vi "Control SCR-1.vi"() -> ()   [LabVIEW 2019]
uses:
  PortConfig.ctl
  <vilib>/Platform/TimedLoop/XDataNode/timing_clust.ctl
  <vilib>/Platform/TimedLoop/XDataNode/nitl_modes.ctl
  <vilib>/Platform/TimedLoop/XDataNode/wakeup.ctl
  <vilib>/Instr/_visa.llb/VISA Configure Serial Port (Instr).vi
  <vilib>/express/express shared/transition.llb/Dynamic To Waveform Array.vi
  <vilib>/express/express signal manip/GetorSetDDTAttributes/Set DDT Attributes/SetT0.vi
  <vilib>/express/express shared/transition.llb/Waveform Array To Dynamic.vi
  <vilib>/express/express signal manip/GetorSetDDTAttributes/Set DDT Attributes/Set DDT Properties.xnode
  <vilib>/platform/TimedLoop/XDataNode/XDataNode.xnode
  <vilib>/Platform/TimedLoop/XDataNode/XDNodeRunTimeDep.lvlib
panel:
  in  "CODIGO DIWO":dbl
  out "Total":dbl format="%#_6f"
  out "Total":dbl(slide) scale=0.0..1500.0
  out "Bobina 4":dbl format="%_3g"
  out "Bobina 0":dbl format="%_3g"
  out "Bobina 8":dbl format="%_3g"
  out "Boolean0":bool
  out "Boolean4":bool
  out "Boolean8":bool
  out "ExeState":string
  out "Next":dbl
  out "ULTIMA":dbl
  in  "Tension en Banco":dbl
  in  "Temperatura en Resistencia":dbl
  out "Temperatura en Bobinas":dbl
  out "E. ECRH":bool
  out "E. Campo":bool
  in  "Stop Button":bool
  out "SECUENCIA FINALIZADA":bool
  out "SECUENCIA INICIADA":bool
  out "Bool0":bool
  out "Bool1":bool
  out "Bool2":bool
  out "Bool3":bool
  out "DESACTIVAR Gas":bool
  out "DESCATIVAR ECRH":bool=TRUE
  out "DESACTIVAR Campo":bool=TRUE
  out "ACTIVAR Diagnosticos":bool=TRUE
  out "ACTIVAR ECRH":bool=TRUE
  out "ACTIVAR Campo":bool=TRUE
  out "Presion":dbl
  out "IG Filament Status":string
  out "Presion Normal":bool
  in  "TD [ms]":dbl
  out "Sistema de Inyeccion de Gas":bool
  out "Diagnosticos":bool
  out "Sistema de ECRH":bool
  out "Sistema de Vacío":bool
  out "Sistema de Potencia":bool
  out "Potencia ECRH":dbl
  out "DESCARGA":bool
  out "SP Fuera de Rango":bool
  out "TC Fuera de Rango":bool
  in  "TC [ms]":dbl
  out "TE1+ TE1 Fuera de Rango":bool
  out "Flujo Aisladores":bool
  in  "Set de Potencia":dbl format="%#_3f"
  out "Fuera de Rango":bool
  out "Rango Normal":bool
  out "P. SET":dbl(knob) scale=0.0..2000.0
  in  "OFF-ON":bool
  out "Boolean":bool
  in  "Secuencia de Descarga":bool
  in  "SP [SCCM]":dbl
  in  "TE1 [ms]":dbl
  in  "TE2 [ms]":dbl
  out "Cuenta C":i32
  out "Iteration Duration A":i64
  out "Iteration Duration B":i64
  out "Iteration Duration C":i64
  out "Iteration Duration D":i64
  out "ACTIVAR Gas":bool
  out "SP1":dbl format="%#_6f"
  out "MFC":dbl format="%#_6f"
  out "Flujo":dbl(knob) scale=0.0..20.0
  out "IG":dbl format="%#_6e"
  out "CG2":dbl format="%#_6e"
  out "CG1":dbl format="%#_6e"
  out "P. Forward":dbl(slide) scale=0.0..1500.0
  out "Forward":dbl format="%#_6f"
  out "P. Reflected":dbl(slide) scale=0.0..1500.0
  out "Reflected":dbl format="%#_6f"
  out "Corriente":dbl(knob) scale=0.0..1000.0
  out "Corriente":dbl format="%#_6f"
  in  "MFC":refnum<visa-resource-name>="COM11"
  in  "IonGauge":refnum<visa-resource-name>="COM12"
  in  "Nombre de Archivo":string="SCR-1_TEST.txt"
  in  "Error In":errorcluster
  out "Cuenta B":i32
  out "Cuenta A":i32
  out "Cuenta D":i32
  out "SECUENCIA":bool caption="Boolean"
  out "INYECCION DE GAS":bool caption="Boolean"
  out "DATOS":bool caption="Boolean"
  out "SEGURIDAD":bool caption="Boolean"
  in  "TG 2":i64=5
  in  "TG 1":i64=5
  # "INDICADORES"
  # "CONFIGURACION"
  # "PARAMETROS DE EXPERIMENTO"
  # "CALENTAMIENTO ECRH"
  # "INYECCION DE GAS"
  # "CAMPO MAGNETICO"
  # "MAGNETRON 2kW"
  # "DISPARO DE DIAGNOSTICOS"
  # "GENERACION DE VACIO"
  # "PARAMETROS INICIALES"
  # "Configuracion"
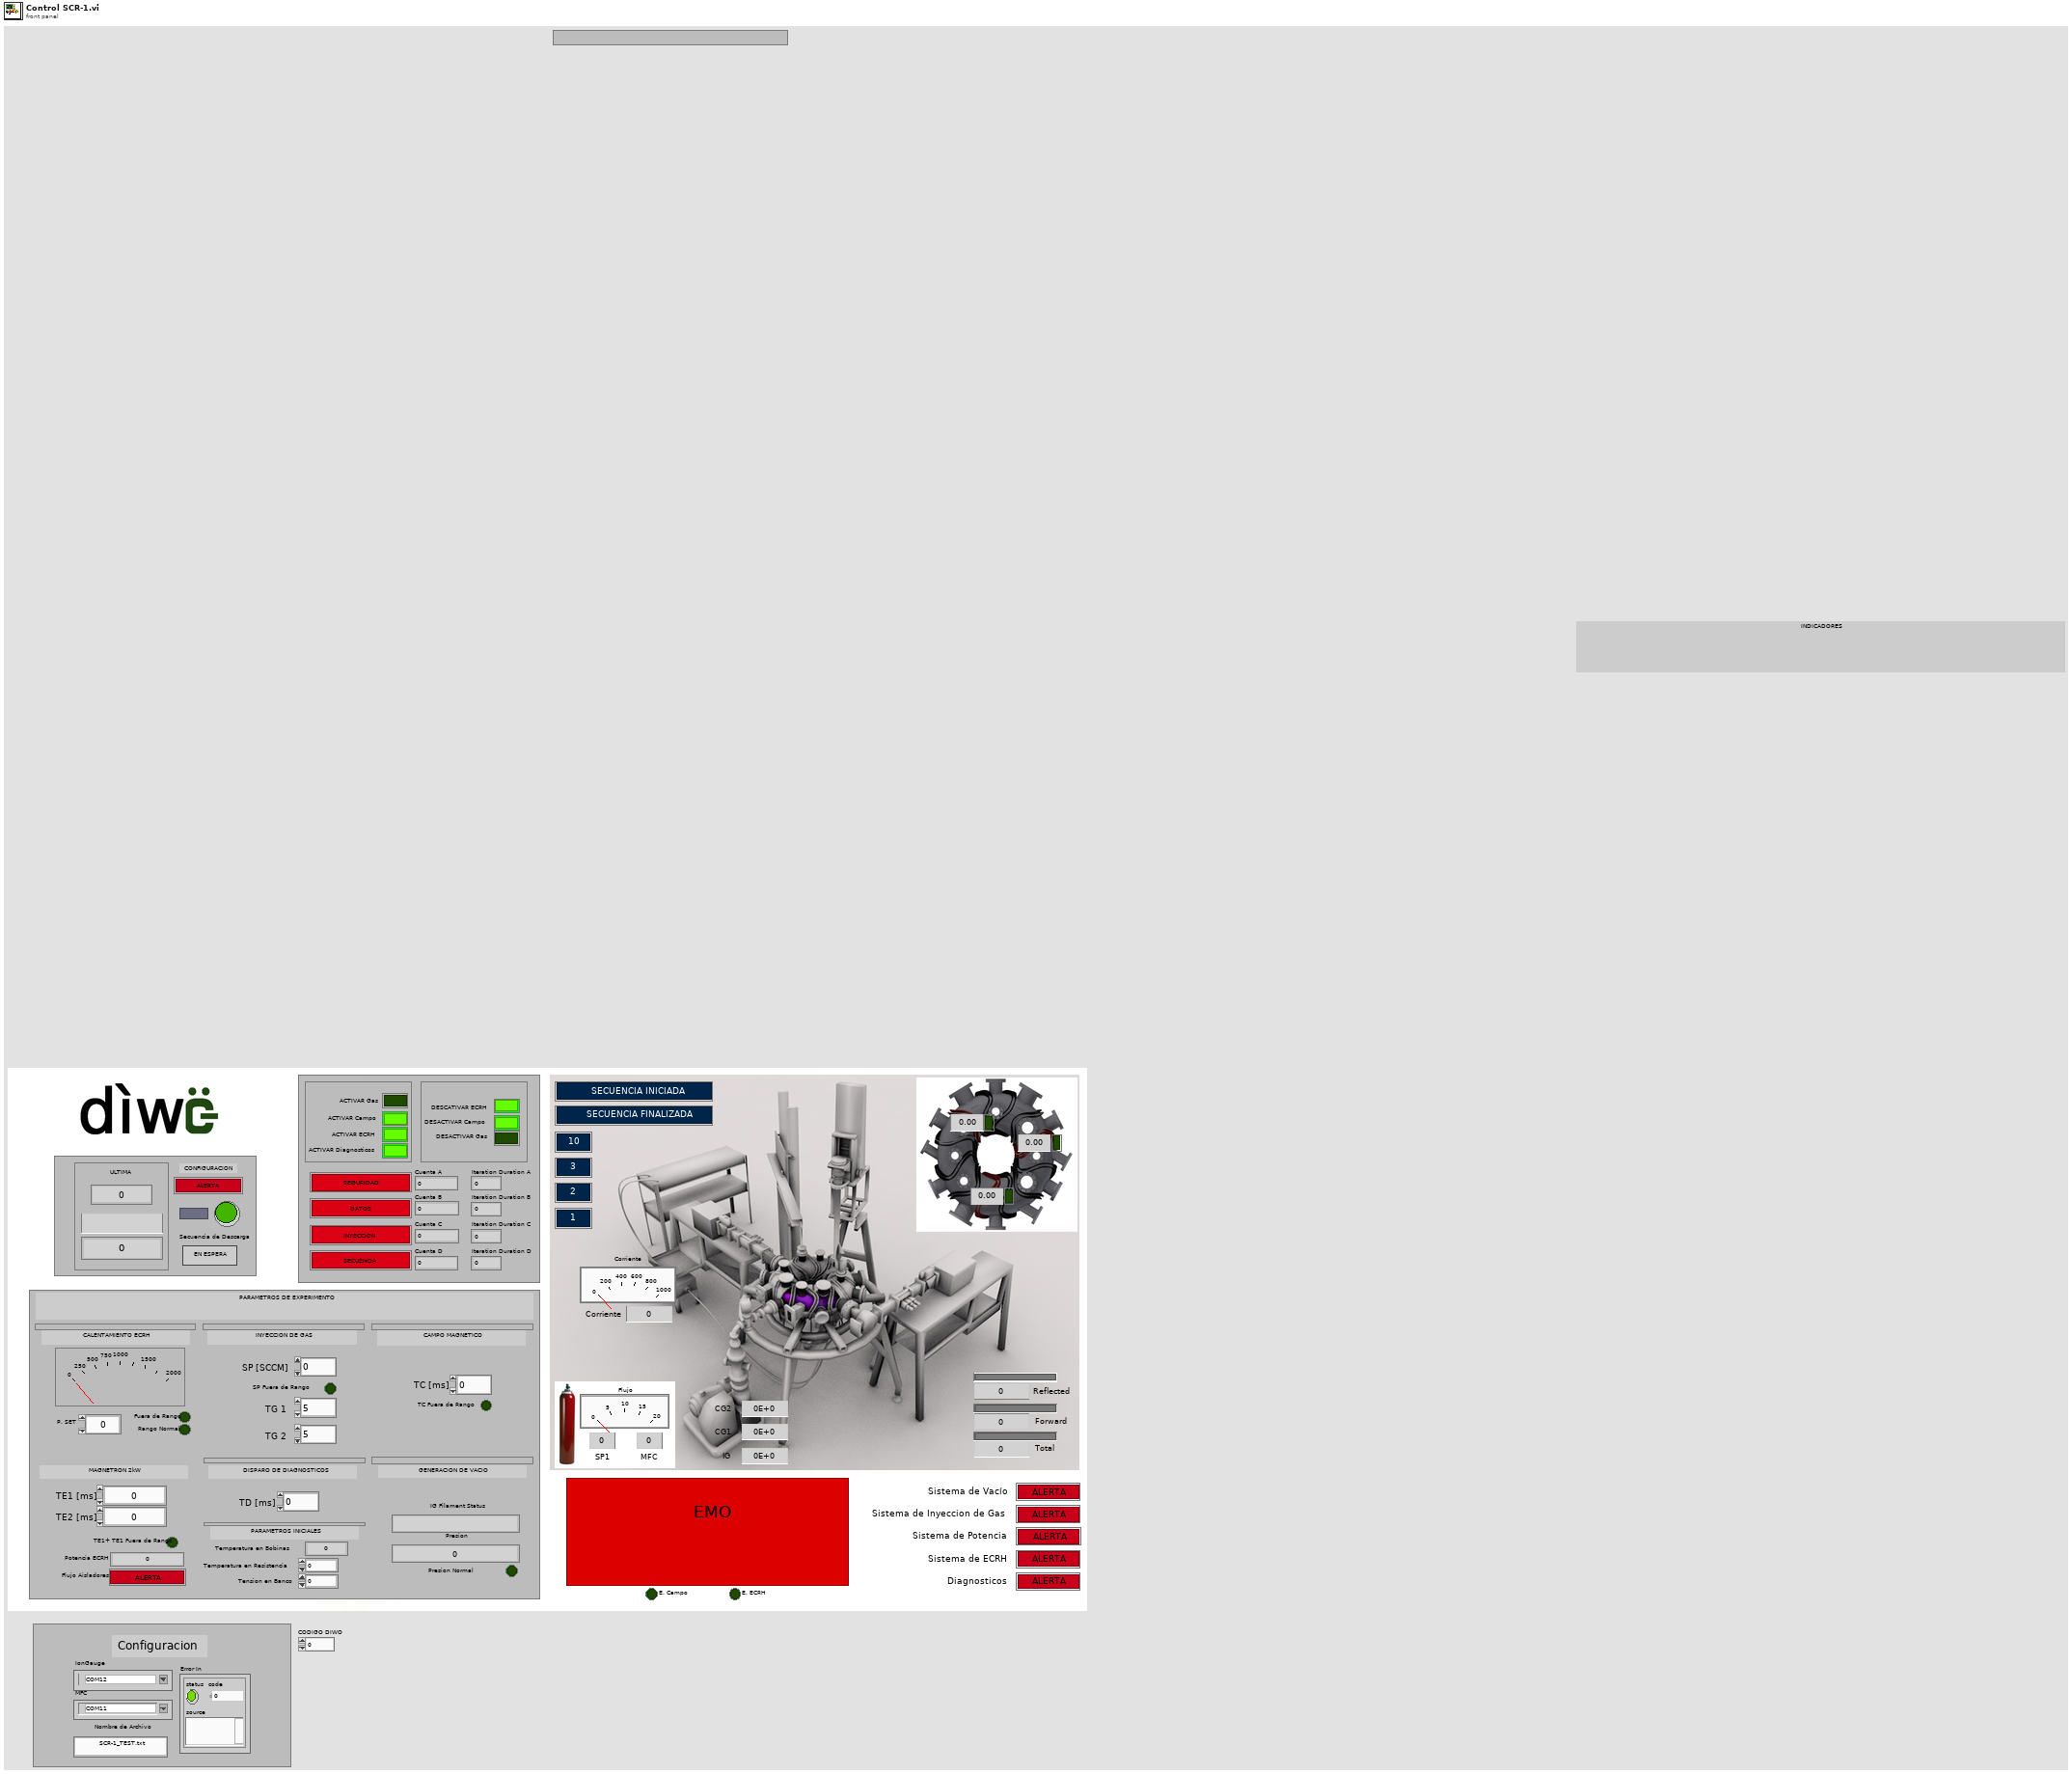
[diagram p1: front panel]
types:
  T1 = typedef "PortConfig.ctl" = cluster{"baud rate":u32, "data bits":u16, "parity":enum16{"None", "Odd", "Even", "Mark", "Space"}, "stop bits":u16}
  T2 = cluster{"VISA resource name out":refnum<visa-resource-name>, "error out":errorcluster, "VISA resource name out":refnum<visa-resource-name>, "error out":errorcluster}
  T3 = cluster{"TD [ms]":dbl, "Set de Potencia":dbl, "TE2 [ms]":dbl, "TE1 [ms]":dbl, "TC [ms]":dbl, "SP [SCCM] ":dbl}
  T4 = typedef "XDNodeRunTimeDep.lvlib/timing_clust.ctl" = cluster{"Expected End [f-1]":u64, "Actual End [f-1]":u64, "Finished Late? [f-1]":bool, "Expected End [i-1]":u64, "Actual End [i-1]":u64, "Finished Late? [i-1]":bool, "Expected Start [i]":u64, "Actual Start [i]":u64, "Expected Start [f]":u64, "Actual Start [f]":u64, "Source Name":string, "Structure Name":string, "Period":i64, "Deadline":i64, "Offset":i64, "Start":i64, "Priority":i32, "Timeout":i32, "Mode":T5, "Wakeup Reason":T6, "Error":errorcluster, "Source Type":string, "Secondary Source Type":string, "Global End Time":u64, "Global Start Time":u64, "Frame Duration":u64, "Iteration Duration":u64, "Assigned CPU":i32, "I/O Scan Engine Mode":u32}
  T5 = typedef "XDNodeRunTimeDep.lvlib/nitl_modes.ctl" = enum32{"No Change", "Process missed periods, maintain original phase", "Discard missed periods, maintain original phase", "Process missed periods, ignore original phase", "Discard missed periods, ignore original phase"}
  T6 = typedef "XDNodeRunTimeDep.lvlib/wakeup.ctl" = enum32{"Normal", "Aborted", "Asynchronous wakeup", "Timing source error", "Timed loop error", "Timeout"}
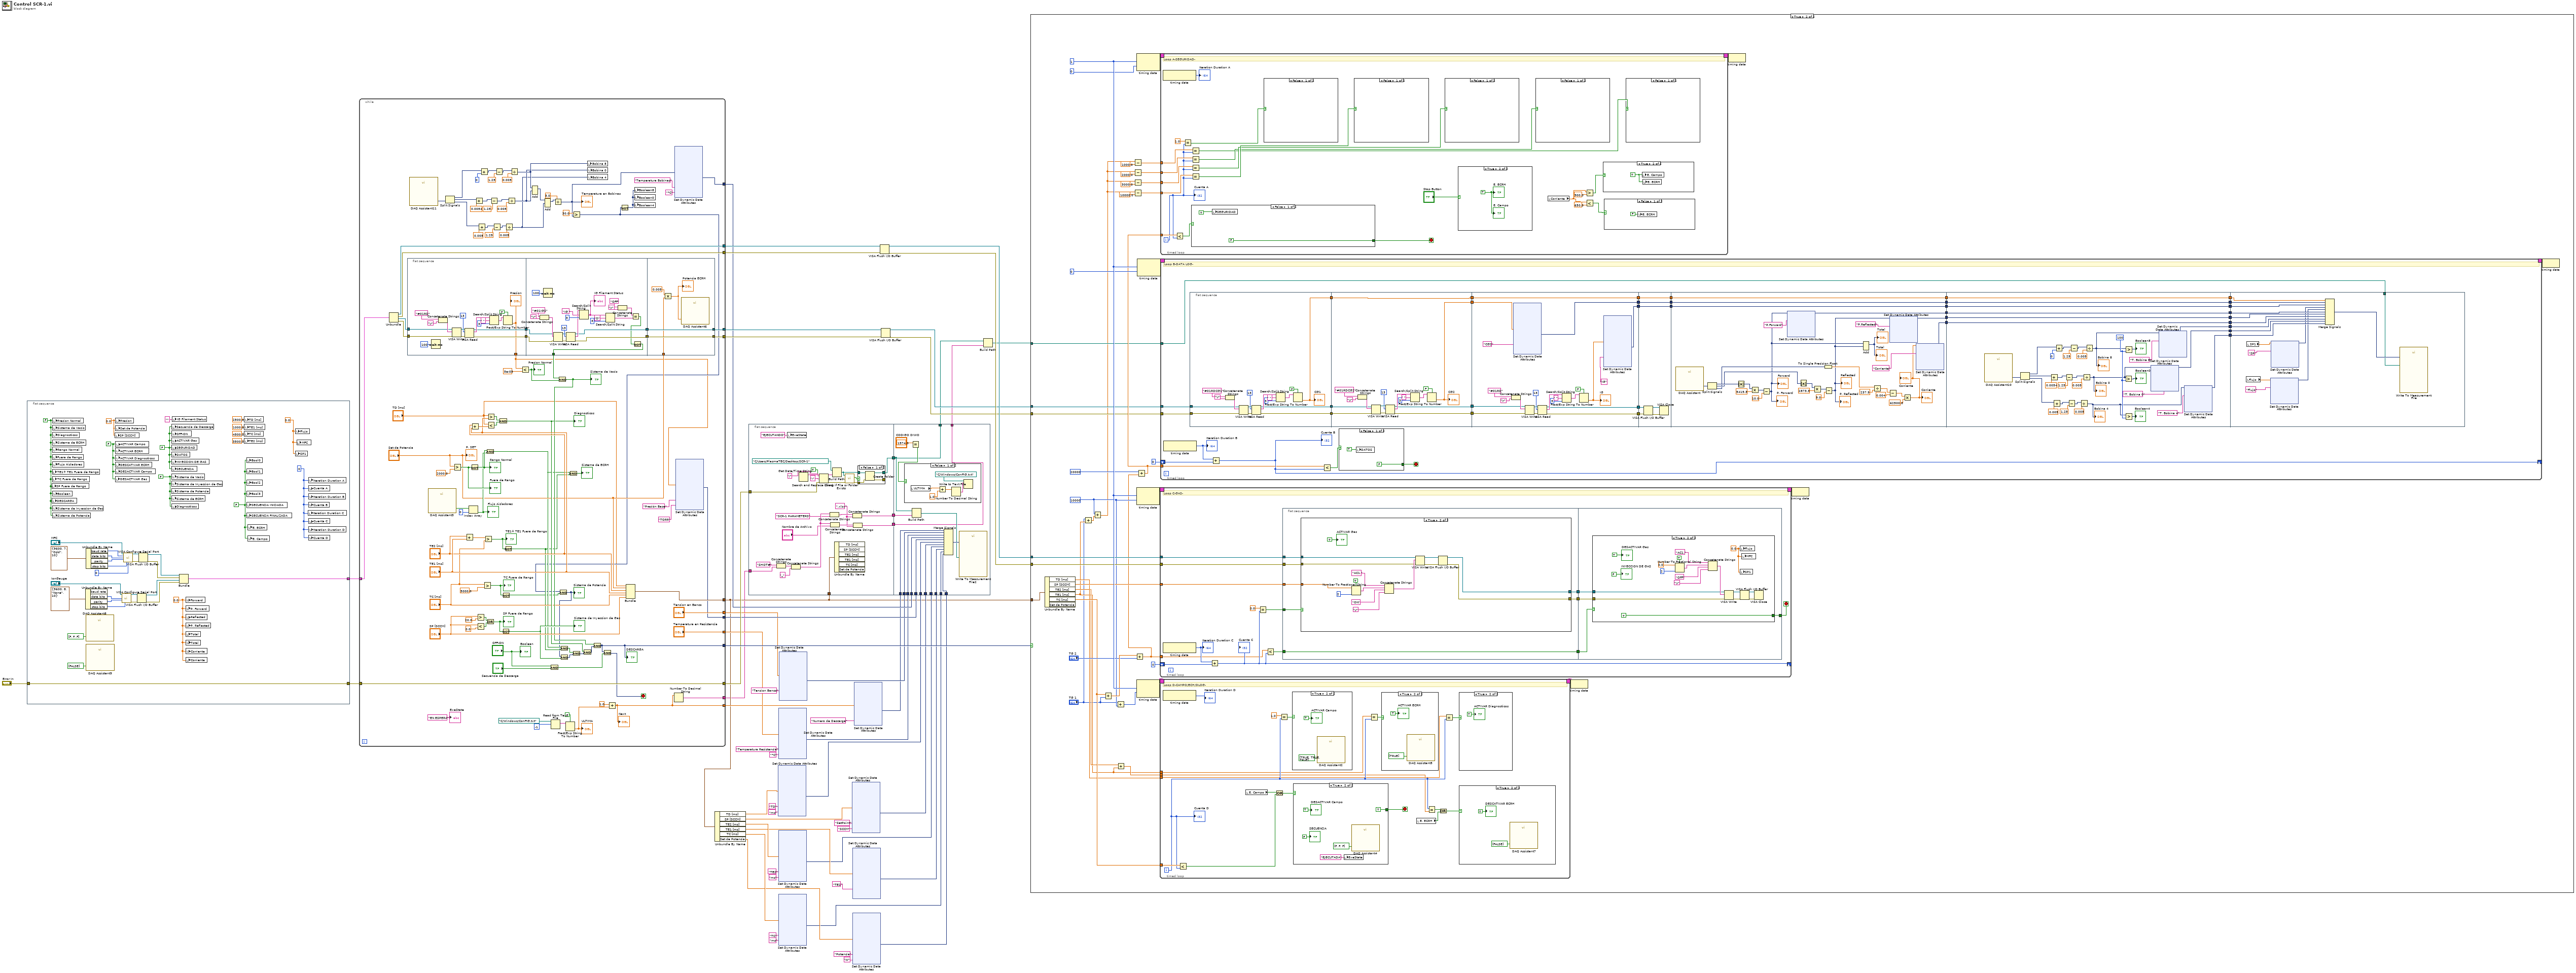
[diagram p0: block diagram]
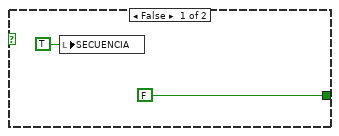
[diagram p9: hidden frame]
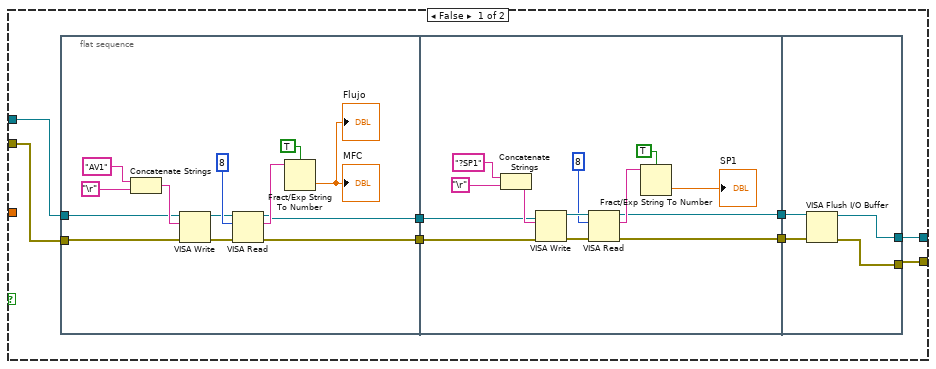
[diagram p10: hidden frame]
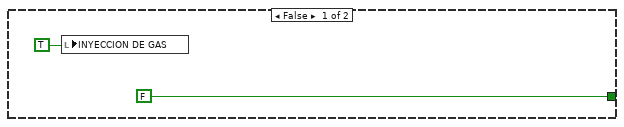
[diagram p11: hidden frame]
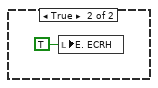
[diagram p12: hidden frame]
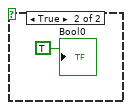
[diagram p15: hidden frame]
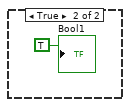
[diagram p16: hidden frame]
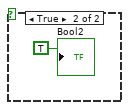
[diagram p17: hidden frame]
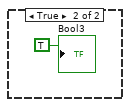
[diagram p18: hidden frame]
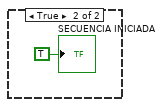
[diagram p19: hidden frame]
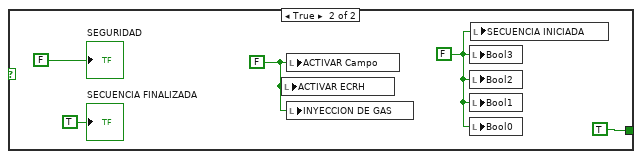
[diagram p20: hidden frame]
diagram:
  n1 = flat-sequence {
    tunnel: [w94] -> w52
    tunnel: "Error In" -> [w94]
    tunnel: [w80] -> w48
    frame #0 {
      w57 = 0.0 ("Forward")
      w62 = 0.0 ("SetPoint")
      w58 = i64 0 ("Iteration Duration C")
      w61 = FALSE ("SECUENCIA INICIADA")
      w63 = FALSE ("CAMPO ON")
      w69 = 0.0 ("Presion")
      w78 = FALSE ("Presion Normal")
      w93 = FALSE ("Sistema de Vacío")
      w64 = FALSE ("SEGURIDAD")
      n2 = local write "SP Fuera de Rango"(w78) -> ()
      n3 = local write "DESCARGA"(w78) -> ()
      n4 = local write "TE1+ TE1 Fuera de Rango"(w78) -> ()
      n5 = local write "TC Fuera de Rango"(w78) -> ()
      n6 = local write "Presion Normal"(w78) -> ()
      n7 = local write "Sistema de Vacío"(w78) -> ()
      n8 = local write "Diagnosticos"(w78) -> ()
      n9 = local write "Sistema de ECRH"(w78) -> ()
      n10 = local write "Rango Normal"(w78) -> ()
      n11 = local write "Fuera de Rango"(w78) -> ()
      n12 = local write "Flujo Aisladores"(w78) -> ()
      n13 = local write "Boolean"(w78) -> ()
      n14 = local write "Sistema de Inyeccion de Gas"(w78) -> ()
      n15 = local write "Sistema de Potencia"(w78) -> ()
      n16 = Unbundle By Name(T1 {"baud rate"=9600, "data bits"=8, "parity"=enum."None", "stop bits"=10} ("Serial Settings")) -> ("data bits"=w82:u16, "parity"=w81:enum16{"None", "Odd", "Even", "Mark", "Space"}, "stop bits"=w83:u16)  [unwired: 1 out]
      n17 = call "DAQ Assistant8"("data"=bool[] [FALSE, FALSE, FALSE]) -> ()  [unwired: 17 in, 2 out]
      n18 = Unbundle By Name(T1 {"baud rate"=9600, "data bits"=7, "parity"=enum."Odd", "stop bits"=10} ("Serial Settings")) -> ("baud rate"=w90:u32, "data bits"=w86:u16, "parity"=w85:enum16{"None", "Odd", "Even", "Mark", "Space"}, "stop bits"=w87:u16)
      n19 = call "DAQ Assistant9"("data"=bool[] [FALSE]) -> ()  [unwired: 17 in, 2 out]
      n20 = local write "SP [SCCM]"(w69) -> ()
      n21 = local write "DESACTIVAR Gas"(w63) -> ()
      n22 = local write "Presion"(w69) -> ()
      n23 = local write "Set de Potencia"(w69) -> ()
      n24 = local write "ACTIVAR Campo"(w63) -> ()
      n25 = local write "ACTIVAR ECRH"(w63) -> ()
      n26 = local write "ACTIVAR Diagnosticos"(w63) -> ()
      n27 = local write "DESCATIVAR ECRH"(w63) -> ()
      n28 = local write "DESACTIVAR Campo"(w63) -> ()
      n29 = call-poly "VISA Configure Serial Port"("VISA resource name"="IonGauge", "data bits (8)"=w82, "parity (0:none)"=w81, "stop bits (10: 1 bit)"=w83) -> ("VISA resource name out"=w72:refnum<visa-resource-name>, "error out"=w71:errorcluster)  [unwired: 10 in]
      n30 = call-poly "VISA Configure Serial Port"("VISA resource name"="MFC", "baud rate (9600)"=w90, "data bits (8)"=w86, "parity (0:none)"=w85, "stop bits (10: 1 bit)"=w87, "flow control (0:none)"=0) -> ("VISA resource name out"=w77:refnum<visa-resource-name>, "error out"=w75:errorcluster)  [unwired: 8 in]
      n31 = VISA Flush I/O Buffer(VISA resource name=w72, error in (no error)=w71) -> (VISA resource name out=w73:refnum<visa-resource-name>, error out=w70:errorcluster)  [unwired: 1 in]
      n32 = VISA Flush I/O Buffer(VISA resource name=w77, error in (no error)=w75) -> (VISA resource name out=w76:refnum<visa-resource-name>, error out=w74:errorcluster)  [unwired: 1 in]
      n33 = local write "Secuencia de Descarga"(w64) -> ()
      n34 = local write "OFF-ON"(w64) -> ()
      n35 = local write "ACTIVAR Gas"(w64) -> ()
      n36 = local write "SEGURIDAD"(w64) -> ()
      n37 = local write "DATOS"(w64) -> ()
      n38 = local write "INYECCION DE GAS"(w64) -> ()
      n39 = local write "SECUENCIA"(w64) -> ()
      n40 = local write "Sistema de Vacío"(w93) -> ()
      n41 = local write "Sistema de Inyeccion de Gas"(w93) -> ()
      n42 = local write "Sistema de Potencia"(w93) -> ()
      n43 = local write "Sistema de ECRH"(w93) -> ()
      n44 = local write "Diagnosticos"(w93) -> ()
      n45 = local write "IG Filament Status"("" ("IG Filament Status")) -> ()
      n46 = Bundle("VISA resource name out"=w76, "error out"=w74, "VISA resource name out"=w73, "error out"=w70) -> (w80:T2)  [unwired: 1 in]
      n47 = local write "Forward"(w57) -> ()
      n48 = local write "P. Forward"(w57) -> ()
      n49 = local write "Reflected"(w57) -> ()
      n50 = local write "P. Reflected"(w57) -> ()
      n51 = local write "Total"(w57) -> ()
      n52 = local write "Total"(w57) -> ()
      n53 = local write "Corriente"(w57) -> ()
      n54 = local write "Corriente"(w57) -> ()
      n55 = local write "TD [ms]"(2500.0 ("TD [ms]")) -> ()
      n56 = local write "TE1 [ms]"(1000.0 ("TE1 [ms]")) -> ()
      n57 = local write "TC [ms]"(4500.0 ("TC [ms]")) -> ()
      n58 = local write "TE2 [ms]"(3500.0 ("TE2 [ms]")) -> ()
      n59 = local write "Bool0"(w61) -> ()
      n60 = local write "Bool1"(w61) -> ()
      n61 = local write "Bool2"(w61) -> ()
      n62 = local write "Bool3"(w61) -> ()
      n63 = local write "SECUENCIA INICIADA"(w61) -> ()
      n64 = local write "SECUENCIA FINALIZADA"(w61) -> ()
      n65 = local write "E. ECRH"(w61) -> ()
      n66 = local write "E. Campo"(w61) -> ()
      n67 = local write "Flujo"(w62) -> ()
      n68 = local write "SP1"(w62) -> ()
      n69 = local write "MFC"(w62) -> ()
      n70 = local write "Iteration Duration C"(w58) -> ()
      n71 = local write "Iteration Duration A"(w58) -> ()
      n72 = local write "Cuenta A"(w58) -> ()
      n73 = local write "Iteration Duration B"(w58) -> ()
      n74 = local write "Cuenta B"(w58) -> ()
      n75 = local write "Cuenta C"(w58) -> ()
      n76 = local write "Iteration Duration D"(w58) -> ()
      n77 = local write "Cuenta D"(w58) -> ()
    }
  }
  n78 = while {
    tunnel: [w154] -> w56
    tunnel: w52 -> [w198]
    tunnel: [w198] -> w51
    tunnel: [w178] -> w4
    tunnel: w48 -> [w170]
    tunnel: [w163] -> w47
    tunnel: [w162] -> w46
    tunnel: [w167] -> w45
    tunnel: [w166] -> w44
    tunnel: [w98] -> w32
    tunnel: ["Tension en Banco"] -> w36
    tunnel: ["Temperatura en Resistencia"] -> w34
    tunnel: [w104] -> w39
    tunnel: [w106] -> w37
    tunnel: [w97] -> w2
    stop <- w155 stop-if-true
    n79 = Unbundle(w170) -> ("VISA resource name out"=w167:refnum<visa-resource-name>, "error out"=w166:errorcluster, "VISA resource name out"=w169:refnum<visa-resource-name>, "error out"=w168:errorcluster)
    n80 = flat-sequence {
      tunnel: w169 -> [w238]
      tunnel: w168 -> [w237]
      tunnel: [w240] -> w165
      tunnel: [w239] -> w164
      tunnel: [w236] -> w95
      tunnel: w165 -> [w258]
      tunnel: w164 -> [w259]
      tunnel: [w252] -> w96
      tunnel: [w257] -> w152
      tunnel: [w256] -> w151
      tunnel: [w278] -> w162
      tunnel: [w279] -> w163
      tunnel: w152 -> [w279]
      tunnel: w151 -> [w278]
      tunnel: "Set de Potencia" -> [w276]
      frame #0 {
        n81 = Wait (ms)(milliseconds to wait=u32 100) -> ()  [unwired: 1 out]
        n82 = Concatenate Strings("#01RD", "\r") -> (w247:string)
        n83 = VISA Write(VISA resource name=w238, write buffer=w247, error in (no error)=w237) -> (VISA resource name out=w250:refnum<visa-resource-name>, error out=w251:errorcluster)  [unwired: 1 out]
        n84 = VISA Read(VISA resource name=w250, byte count=13, error in (no error)=w251) -> (VISA resource name out=w240:refnum<visa-resource-name>, read buffer=w241:string, error out=w239:errorcluster)  [unwired: 1 out]
        n85 = Search/Split String(string=w241, search string/char (-)=" ", offset (0)=3) -> (match + rest of string=w245:string)  [unwired: 2 out]
        n86 = Fract/Exp String To Number(use system decimal point (T)=FALSE, string=w245) -> (number=w236:dbl)  [unwired: 2 in, 1 out]
        "Presion" <- w236
      }
      frame #1 {
        n87 = Concatenate Strings("#01IGS", "\r") -> (w265:string)
        n88 = Wait (ms)(milliseconds to wait=u32 100) -> ()  [unwired: 1 out]
        n89 = VISA Write(VISA resource name=w258, write buffer=w265, error in (no error)=w259) -> (VISA resource name out=w261:refnum<visa-resource-name>, error out=w255:errorcluster)  [unwired: 1 out]
        n90 = VISA Read(VISA resource name=w261, byte count=13, error in (no error)=w255) -> (VISA resource name out=w257:refnum<visa-resource-name>, read buffer=w260:string, error out=w256:errorcluster)  [unwired: 1 out]
        n91 = Search/Split String(string=w260, search string/char (-)="IG ", offset (0)=3) -> (match + rest of string=w274:string)  [unwired: 2 out]
        "IG Filament Status" <- w274
        n92 = Search/Split String(string=w274, search string/char (-)="O", offset (0)=3) -> (match + rest of string=w273:string)  [unwired: 2 out]
        n93 = Concatenate Strings("OFF", "\r") -> (w272:string)
        n94 = Equal?(x=w272, y=w273) -> (x = y?=w253:bool)
        n95 = Not(x=w253) -> (.not. x?=w252:bool)
      }
      frame #2 {
        n96 = Multiply(x=0.005, y=w276) -> (x*y=w275:dbl)
        "Potencia ECRH" <- w275
        n97 = call "DAQ Assistant6"("data"=w275) -> ()  [unwired: 17 in, 2 out]
      }
    }
    n98 = call "DAQ Assistant11"() -> ("data"=w123:dynamicdata)  [unwired: 17 in, 2 out]
    n99 = call "DAQ Assistant3"() -> ("data"=w180:bool[])  [unwired: 17 in, 2 out]
    n100 = Split Signals(w123) -> (w133:dynamicdata, w134:dynamicdata, w135:dynamicdata)  [unwired: 3 in]
    n101 = Greater?(x="Set de Potencia", y=2000.0 ("x")) -> (0:w183:bool)
    "Fuera de Rango" <- w183
    n102 = Add(x="TE2 [ms]", y="TE1 [ms]") -> (x+y=w188:dbl)
    n103 = Index Array(array=w180, index=0) -> (element=w182:bool)
    "Flujo Aisladores" <- w182
    n104 = Not(x=w183) -> (.not. x?=w184:bool)
    "Rango Normal" <- w184
    n105 = Add(x="TE2 [ms]", y="TE1 [ms]") -> (x+y=w174:dbl)
    n106 = Add(x=w134, y=0.0054) -> (x+y=w137:dynamicdata)
    n107 = Greater?(x="SP [SCCM]", y=20.0) -> (0:w195:bool)
    n108 = Less?(x="SP [SCCM]", y=0.0) -> (x < y?=w194:bool)
    n109 = Add(x=w135, y=0.005) -> (x+y=w136:dynamicdata)
    n110 = Add(x=w133, y=0) -> (x+y=w138:dynamicdata)
    n111 = Greater?(x="TC [ms]", y=5000.0) -> (0:w191:bool)
    "TC Fuera de Rango" <- w191
    n112 = Greater?(x=w188, y="TC [ms]") -> (0:w189:bool)
    "TE1+ TE1 Fuera de Rango" <- w189
    n113 = And(x=w184, y=w182) -> (x .and. y?=w147:bool)
    n114 = Or(x=w195, y=w194) -> (x .or. y?=w196:bool)
    "SP Fuera de Rango" <- w196
    n115 = Greater?(x="TD [ms]", y="TE1 [ms]") -> (0:w176:bool)
    n116 = Less?(x="TD [ms]", y=w174) -> (x < y?=w175:bool)
    n117 = Subtract(x=w137, y=1.25) -> (x-y=w126:dynamicdata)
    n118 = Subtract(x=w136, y=1.25) -> (x-y=w130:dynamicdata)
    n119 = Subtract(x=w138, y=1.25) -> (x-y=w121:dynamicdata)
    n120 = And(x=w176, y=w175) -> (x .and. y?=w153:bool)
    "Diagnosticos" <- w153
    n121 = Not(x=w196) -> (.not. x?=w177:bool)
    "Sistema de Inyeccion de Gas" <- w177
    n122 = Not(x=w191) -> (.not. x?=w115:bool)
    n123 = Not(x=w189) -> (.not. x?=w146:bool)
    n124 = Divide(x=w130, y=0.005) -> (x/y=w111:dynamicdata)
    n125 = Divide(x=w126, y=0.005) -> (x/y=w112:dynamicdata)
    n126 = Divide(x=w121, y=0.005) -> (x/y=w113:dynamicdata)
    n127 = Less?(x=w95, y=5e-05 ("x")) -> (x < y?=w161:bool)
    "Presion Normal" <- w161
    n128 = Add(1:w112, 2:w113) -> (0:w119:dynamicdata)  [unwired: 1 in, 1 out]
    n129 = Add(1:w111, 2:w119) -> (0:w118:dynamicdata)  [unwired: 1 in, 1 out]
    n130 = And(x="OFF-ON", y="Secuencia de Descarga") -> (x .and. y?=w156:bool)
    n131 = Read from Text File(file (use dialog)=path "C:/Windows/ConFIG.txt", count=-1) -> (text=w144:string)  [unwired: 2 in, 3 out]
    n132 = Divide(x=w118, y=3.0) -> (x/y=w103:dynamicdata)
    "Temperatura en Bobinas" <- w103
    n133 = And(x=w96, y=w161) -> (x .and. y?=w159:bool)
    "Sistema de Vacío" <- w159
    n134 = And(x=w147, y=w146) -> (x .and. y?=w171:bool)
    n135 = Fract/Exp String To Number(use system decimal point (T)=FALSE, string=w144) -> (number=w141:dbl)  [unwired: 2 in, 1 out]
    "ULTIMA" <- w141
    n136 = And(x=w147, y=w146) -> (x .and. y?=→"Sistema de ECRH":bool)
    n137 = Greater?(x=30.0 ("y"), y=w103) -> (0:w109:dynamicdata)
    n138 = And(x=w109, y=w115) -> (x .and. y?=w116:dynamicdata)
    "Sistema de Potencia" <- w116
    n139 = And(x=w116, y=w177) -> (x .and. y?=w197:dynamicdata)
    n140 = And(x=w171, y=w197) -> (x .and. y?=w158:dynamicdata)
    n141 = And(x=w153, y=w158) -> (x .and. y?=w157:dynamicdata)
    n142 = local write "Bobina 8"(w113) -> ()
    n143 = local write "Bobina 0"(w112) -> ()
    n144 = local write "Bobina 4"(w111) -> ()
    n145 = And(x=w159, y=w157) -> (x .and. y?=w154:dynamicdata)
    "DESCARGA" <- w154
    n146 = And(x=w154, y=w156) -> (x .and. y?=w155:dynamicdata)
    n147 = Add(x=1.0, y=w141) -> (x+y=w98:dbl)
    "Next" <- w98
    n148 = Not(x=w109) -> (.not. x?=w110:dynamicdata)
    n149 = Bundle("TD [ms]"="TD [ms]", "Set de Potencia"="Set de Potencia", "TE2 [ms]"="TE2 [ms]", "TE1 [ms]"="TE1 [ms]", "TC [ms]"="TC [ms]", "SP [SCCM]"="SP [SCCM]") -> (w178:T3)  [unwired: 1 in]
    n150 = local write "Boolean8"(w110) -> ()
    n151 = local write "Boolean0"(w110) -> ()
    n152 = local write "Boolean4"(w110) -> ()
    n153 = Number To Decimal String(number=w98) -> (decimal integer string=w97:string)  [unwired: 1 in]
    n154 = xnode "Set Dynamic Data Attributes"("Signals In"=w103, "Signal Name"="Temperatura Bobinas", "Unit"="°C") -> ("Signals Out"=w104:dynamicdata)  [unwired: 2 in, 1 out]
    n155 = xnode "Set Dynamic Data Attributes"("Signals In"=w95, "Signal Name"="Presión Base", "Unit"="TORR") -> ("Signals Out"=w106:dynamicdata)  [unwired: 2 in, 1 out]
    "P. SET" <- "Set de Potencia"
    "Boolean" <- "OFF-ON"
    "ExeState" <- "EN ESPERA" ("ExeState")
  }
  n156 = Unbundle By Name(w4) -> ("TD [ms]"=w26:dbl, "SP [SCCM]"=w25:dbl, "TE2 [ms]"=w24:dbl, "TE1 [ms]"=w23:dbl, "TC [ms]"=w22:dbl, "Set de Potencia"=w21:dbl)
  n157 = flat-sequence {
    tunnel: w51 -> [w295]
    tunnel: [w294] -> w42
    tunnel: [w288] -> w38
    tunnel: w4 -> [w292]
    tunnel: [w287] -> w3
    tunnel: w2 -> [w286]
    tunnel: w42 -> [w322]
    tunnel: [w322] -> w41
    tunnel: [w313] -> w40
    tunnel: w31 -> [w326]
    tunnel: w35 -> [w325]
    tunnel: w33 -> [w324]
    tunnel: w39 -> [w323]
    tunnel: w38 -> [w320]
    tunnel: w37 -> [w319]
    tunnel: w20 -> [w318]
    tunnel: w19 -> [w317]
    tunnel: w18 -> [w316]
    tunnel: w17 -> [w312]
    tunnel: w16 -> [w315]
    tunnel: w15 -> [w314]
    tunnel: w3 -> [w313]
    frame #0 {
      w289 = ".xlsx" ("string")
      n158 = Concatenate Strings("SHOT#" ("string"), w286) -> (w284:string)
      n159 = local write "ExeState"("EJECUTANDO" ("ExeState")) -> ()
      n160 = Concatenate Strings(w284, "_" ("string")) -> (w282:string)
      n161 = Get Date/Time String() -> (date string=w305:string)  [unwired: 3 in, 1 out]
      n162 = Search and Replace String(replace all?=TRUE ("replace all? (F)"), input string=w305, search string="/", replace string="-" ("replace string (\"\")"), error in=w295) -> (result string=w300:string, error out=w299:errorcluster)  [unwired: 3 in, 2 out]
      n163 = Concatenate Strings(w282, "SCR-1 PARAMETERS" ("name or relative path")) -> (w290:string)
      n164 = Concatenate Strings(w282, "Nombre de Archivo") -> (w291:string)
      n165 = Build Path(base path=path "C:/Users/PlasmaTEC/Desktop/SCR-1" ("path (use dialog)"), name or relative path=w300) -> (appended path=w297:path)
      n166 = Unbundle By Name(w292) -> ()  [unwired: 6 out]
      n167 = call <vilib>:"Check if File or Folder Exists.vi"("error in (no error)"=w299, "path"=w297) -> ("error out"=w296:errorcluster, "file or folder exists?"=w298:bool)  [unwired: 7 in, 1 out]
      n168 = Concatenate Strings(w290, w289) -> (w288:string)
      n169 = Concatenate Strings(w291, w289) -> (w287:string)
      n170 = case shown="False" w298 {
        tunnel: w297 -> [w309 w311]
        tunnel: w296 -> [w308 w310]
        tunnel: [w307 w311] -> w294
        tunnel: [w306 w310] -> _
        frame False {
          n171 = Create Folder(path (use dialog)=w309, error in=w308) -> (created path=w307:path, error out=w306:errorcluster)  [unwired: 1 in, 1 out]
        }
        frame True {
        }
      }
    }
    frame #1 {
      n172 = Equal?(x="CODIGO DIWO", y=1974.0) -> (x = y?=w328:bool)
      n173 = case shown="False" w328 {
        frame False {
          n174 = local read "ULTIMA"() -> (w331:dbl)
          n175 = Add(x=w331, y=1.0) -> (x+y=w333:dbl)
          n176 = Number To Decimal String(number=w333) -> (decimal integer string=w335:string)  [unwired: 1 in]
          n177 = Write to Text File(file (use dialog)=path "C:/Windows/ConFIG.txt", text=w335) -> ()  [unwired: 2 in, 3 out]
        }
        frame True {
        }
      }
      n178 = Build Path(base path=w322, name or relative path=w320) -> (appended path=w321:path)
      n179 = Merge Signals(w326, w325, w324, w323, w319, w318, w317, w316, w312, w315, w314) -> (w327:dynamicdata)
      n180 = call "Write To Measurement File2"("Signals"=w327, "Filename"=w321) -> ()  [unwired: 15 in, 3 out]
    }
  }
  n181 = xnode "Set Dynamic Data Attributes"("Signals In"=w26, "Signal Name"="TD", "Unit"="ms") -> ("Signals Out"=w20:dynamicdata)  [unwired: 2 in, 1 out]
  n182 = xnode "Set Dynamic Data Attributes"("Signals In"=w24, "Signal Name"="TE2", "Unit"="ms") -> ("Signals Out"=w18:dynamicdata)  [unwired: 2 in, 1 out]
  n183 = xnode "Set Dynamic Data Attributes"("Signals In"=w22, "Signal Name"="TC", "Unit"="ms") -> ("Signals Out"=w16:dynamicdata)  [unwired: 2 in, 1 out]
  n184 = xnode "Set Dynamic Data Attributes"("Signals In"=w34, "Signal Name"="Temperatura Resistencia", "Unit"="°C") -> ("Signals Out"=w33:dynamicdata)  [unwired: 2 in, 1 out]
  n185 = xnode "Set Dynamic Data Attributes"("Signals In"=w36, "Signal Name"="Tension Banco") -> ("Signals Out"=w35:dynamicdata)  [unwired: 2 in, 1 out]
  n186 = xnode "Set Dynamic Data Attributes"("Signals In"=w25, "Signal Name"="SetPoint", "Unit"="SCCM") -> ("Signals Out"=w19:dynamicdata)  [unwired: 2 in, 1 out]
  n187 = xnode "Set Dynamic Data Attributes"("Signals In"=w23, "Signal Name"="TE1") -> ("Signals Out"=w17:dynamicdata)  [unwired: 3 in, 1 out]
  n188 = xnode "Set Dynamic Data Attributes"("Signals In"=w21, "Signal Name"="Potencia", "Unit"="W") -> ("Signals Out"=w15:dynamicdata)  [unwired: 2 in, 1 out]
  n189 = xnode "Set Dynamic Data Attributes"("Signals In"=w32, "Signal Name"="Numero de Descarga") -> ("Signals Out"=w31:dynamicdata)  [unwired: 2 in, 1 out]
  n190 = VISA Flush I/O Buffer(VISA resource name=w45, error in (no error)=w44) -> (VISA resource name out=w55:refnum<visa-resource-name>, error out=w54:errorcluster)  [unwired: 1 in]
  n191 = VISA Flush I/O Buffer(VISA resource name=w47, error in (no error)=w46) -> (VISA resource name out=w50:refnum<visa-resource-name>, error out=w49:errorcluster)  [unwired: 1 in]
  n192 = Build Path(base path=w41, name or relative path=w40) -> (appended path=w43:path)
  n193 = case shown="True" w56 {
    tunnel: w43 -> [_ w362]
    tunnel: w50 -> [_ w361]
    tunnel: w49 -> [_ w360]
    tunnel: w55 -> [_ w359]
    tunnel: w54 -> [_ w358]
    tunnel: w4 -> [_ w355]
    frame False {
    }
    frame True {
      w348 = 10000
      w370 = 1
      n194 = Unbundle By Name(w355) -> ("TD [ms]"=w352:dbl, "SP [SCCM]"=w353:dbl, "TE2 [ms]"=w351:dbl, "TE1 [ms]"=w347:dbl, "TC [ms]"=w354:dbl)  [unwired: 1 out]
      n195 = Add(x="TG 1", y=w347) -> (x+y=w349:dbl)
      n196 = Add(x=w348, y=w349) -> (x+y=w340:dbl)
      n197 = Add(x=w354, y="TG 1") -> (x+y=w366:dbl)
      n198 = Add(x="TG 1", y=w348) -> (x+y=w367:i64)
      n199 = Add(x=w351, y=w347) -> (x+y=w350:dbl)
      n200 = Subtract(x=w340, y=1000.0) -> (x-y=w345:dbl)
      n201 = Subtract(x=w340, y=2000.0) -> (x-y=w344:dbl)
      n202 = Subtract(x=w340, y=3000.0) -> (x-y=w343:dbl)
      n203 = Subtract(x=w340, y=10000.0) -> (x-y=w342:dbl)
      n204 = Add(x=w366, y="TG 2") -> (x+y=w336:dbl)
      n205 = node-c288(w370, w348) -> (w374:T4)
      n206 = node-c288(w370, w367) -> (w372:T4)
      n207 = node-c288(w370, 0) -> (w376:T4)
      n208 = node-c288(w370, i64 0 ("Offset")) -> (w378:T4)
      n209 = Add(x=20000, y=w336) -> (x+y=w363:dbl)
      n210 = timed-loop {
        tunnel: w336 -> [w421]
        timing-out: [_] -> w373
        timing: w374 -> [_]
        tunnel: w359 -> [w426]
        tunnel: w358 -> [w425]
        shift-right: [w422] -> _
        shift-left: 0 -> [w428]
        tunnel: w353 -> [w427]
        stop <- w418 stop-if-true
        # "Loop C-GAS-"
        n211 = node-c288() -> (w429:i64)  [unwired: 1 in]
        "Iteration Duration C" <- w429
        n212 = Add(x=w429, y=w428) -> (x+y=w422:i64)
        "Cuenta C" <- w422
        n213 = Equal?(x=0.0, y=w422) -> (x = y?=w430:bool)
        n214 = Less?(x=w421, y=w422) -> (x < y?=w419:bool)
        n215 = flat-sequence {
          tunnel: w430 -> [w438]
          tunnel: w427 -> [w437]
          tunnel: w426 -> [w436]
          tunnel: w425 -> [w435]
          tunnel: [w434] -> w424
          tunnel: [w433] -> w423
          tunnel: [w432] -> w420
          tunnel: w419 -> [w432]
          tunnel: w424 -> [w495]
          tunnel: w423 -> [w494]
          tunnel: w420 -> [w493]
          tunnel: [w492] -> w418
          frame #0 {
            n216 = case shown="True" w438 {
              tunnel: w436 -> [w441 w481]
              tunnel: w435 -> [w442 w480]
              tunnel: w437 -> [_ w479]
              tunnel: [w440 w477] -> w434
              tunnel: [w439 w478] -> w433
              frame False {
                n217 = flat-sequence {
                  tunnel: w441 -> [w451]
                  tunnel: w442 -> [w450]
                  tunnel: [w449] -> w446
                  tunnel: [w448] -> w445
                  tunnel: w446 -> [w464]
                  tunnel: w445 -> [w463]
                  tunnel: [w461] -> w444
                  tunnel: [w460] -> w443
                  tunnel: w444 -> [w476]
                  tunnel: w443 -> [w475]
                  tunnel: [w474] -> w440
                  tunnel: [w473] -> w439
                  frame #0 {
                    n218 = Concatenate Strings("AV1", "\r") -> (w456:string)
                    n219 = VISA Write(VISA resource name=w451, write buffer=w456, error in (no error)=w450) -> (VISA resource name out=w453:refnum<visa-resource-name>, error out=w452:errorcluster)  [unwired: 1 out]
                    n220 = VISA Read(VISA resource name=w453, byte count=8, error in (no error)=w452) -> (VISA resource name out=w449:refnum<visa-resource-name>, read buffer=w459:string, error out=w448:errorcluster)  [unwired: 1 out]
                    n221 = Fract/Exp String To Number(use system decimal point (T)=TRUE, string=w459) -> (number=→"MFC" →"Flujo":dbl)  [unwired: 2 in, 1 out]
                  }
                  frame #1 {
                    n222 = Concatenate Strings("?SP1", "\r") -> (w468:string)
                    n223 = VISA Write(VISA resource name=w464, write buffer=w468, error in (no error)=w463) -> (VISA resource name out=w471:refnum<visa-resource-name>, error out=w472:errorcluster)  [unwired: 1 out]
                    n224 = VISA Read(VISA resource name=w471, byte count=8, error in (no error)=w472) -> (VISA resource name out=w461:refnum<visa-resource-name>, read buffer=w465:string, error out=w460:errorcluster)  [unwired: 1 out]
                    n225 = Fract/Exp String To Number(use system decimal point (T)=TRUE, string=w465) -> (number=→"SP1":dbl)  [unwired: 2 in, 1 out]
                  }
                  frame #2 {
                    n226 = VISA Flush I/O Buffer(VISA resource name=w476, error in (no error)=w475) -> (VISA resource name out=w474:refnum<visa-resource-name>, error out=w473:errorcluster)  [unwired: 1 in]
                  }
                }
              }
              frame True {
                n227 = Number To Fractional String(use system decimal point (T)=TRUE, number=w479, precision (6)=2) -> (F-format string=w490:string)  [unwired: 1 in]
                n228 = Concatenate Strings("AC1,", w490, "ON", "\r") -> (w484:string)
                n229 = VISA Write(VISA resource name=w481, write buffer=w484, error in (no error)=w480) -> (VISA resource name out=w483:refnum<visa-resource-name>, error out=w482:errorcluster)  [unwired: 1 out]
                n230 = VISA Flush I/O Buffer(VISA resource name=w483, error in (no error)=w482) -> (VISA resource name out=w477:refnum<visa-resource-name>, error out=w478:errorcluster)  [unwired: 1 in]
                "ACTIVAR Gas" <- TRUE
              }
            }
          }
          frame #1 {
            n231 = case shown="True" w493 {
              tunnel: [FALSE TRUE] -> w492
              tunnel: w495 -> [_ w500]
              tunnel: w494 -> [_ w499]
              frame False {
                n232 = local write "INYECCION DE GAS"(TRUE ("SECUENCIA")) -> ()
              }
              frame True {
                w498 = 0.0 ("Flujo")
                n233 = Number To Fractional String(use system decimal point (T)=TRUE, number=0.0, precision (6)=2) -> (F-format string=w511:string)  [unwired: 1 in]
                n234 = Concatenate Strings("AC1,", w511, "OFF", "\r") -> (w505:string)
                n235 = VISA Write(VISA resource name=w500, write buffer=w505, error in (no error)=w499) -> (VISA resource name out=w504:refnum<visa-resource-name>, error out=w503:errorcluster)  [unwired: 1 out]
                n236 = VISA Flush I/O Buffer(VISA resource name=w504, error in (no error)=w503) -> (VISA resource name out=w513:refnum<visa-resource-name>, error out=w512:errorcluster)  [unwired: 1 in]
                n237 = local write "Flujo"(w498) -> ()
                n238 = local write "SP1"(w498) -> ()
                n239 = local write "MFC"(w498) -> ()
                n240 = VISA Close(VISA resource name=w513, error in (no error)=w512) -> ()  [unwired: 1 out]
                "INYECCION DE GAS" <- FALSE ("SECUENCIA")
                "DESACTIVAR Gas" <- TRUE
              }
            }
          }
        }
      }
      n241 = timed-loop {
        timing-out: [_] -> w371
        timing: w372 -> [_]
        tunnel: w354 -> [w395]
        tunnel: w347 -> [w387]
        tunnel: w352 -> [w388]
        tunnel: w350 -> [w386]
        i -> [w389]
        stop <- w394 stop-if-true
        # "Loop D-CAMPO/ECH/DLOG-"
        n242 = node-c288() -> (→"Iteration Duration D":i64)  [unwired: 1 in]
        n243 = Less?(x=w395, y=w389) -> (x < y?=w383:bool)
        n244 = local read "E. Campo"() -> (w382:bool)
        n245 = Or(x=w382, y=w383) -> (x .or. y?=w384:bool)
        n246 = Equal?(x=1.0, y=w389) -> (x = y?=w393:bool)
        n247 = case shown="True" w393 {
          frame False {
          }
          frame True {
            n248 = call "DAQ Assistant2"("data"=bool[] [TRUE, TRUE, TRUE]) -> ()  [unwired: 17 in, 2 out]
            "ACTIVAR Campo" <- TRUE
          }
        }
        n249 = case shown="True" w384 {
          tunnel: [FALSE TRUE] -> w394
          frame False {
            n250 = local write "SECUENCIA"(TRUE ("SECUENCIA")) -> ()
          }
          frame True {
            n251 = local write "ExeState"("EJECUTADA" ("ExeState")) -> ()
            n252 = call "DAQ Assistant4"("data"=bool[] [FALSE, FALSE, FALSE]) -> ()  [unwired: 17 in, 2 out]
            "SECUENCIA" <- FALSE ("SECUENCIA")
            "DESACTIVAR Campo" <- TRUE
          }
        }
        n253 = Equal?(x=w387, y=w389) -> (x = y?=w392:bool)
        n254 = case shown="True" w392 {
          frame False {
          }
          frame True {
            n255 = call "DAQ Assistant5"("data"=bool[] [TRUE]) -> ()  [unwired: 17 in, 2 out]
            "ACTIVAR ECRH" <- TRUE
          }
        }
        n256 = local read "E. ECRH"() -> (w379:bool)
        n257 = Equal?(x=w389, y=w386) -> (x = y?=w381:bool)
        n258 = Or(x=w381, y=w379) -> (x .or. y?=w380:bool)
        n259 = Equal?(x=w388, y=w389) -> (x = y?=w391:bool)
        n260 = case shown="True" w391 {
          frame False {
          }
          frame True {
            "ACTIVAR Diagnosticos" <- TRUE
          }
        }
        n261 = case shown="True" w380 {
          frame False {
          }
          frame True {
            n262 = call "DAQ Assistant7"("data"=bool[] [FALSE]) -> ()  [unwired: 17 in, 2 out]
            "DESCATIVAR ECRH" <- TRUE
          }
        }
        "Cuenta D" <- w389
      }
      n263 = timed-loop {
        tunnel: w363 -> [w544]
        timing-out: [_] -> w375
        timing: w376 -> [_]
        tunnel: w345 -> [w540]
        tunnel: w344 -> [w539]
        tunnel: w343 -> [w538]
        tunnel: w342 -> [w537]
        i -> [w535]
        stop <- w542 stop-if-true
        # "Loop A-SEGURIDAD-"
        n264 = node-c288() -> (→"Iteration Duration A":i64)  [unwired: 1 in]
        n265 = Less?(x=w544, y=w535) -> (x < y?=w543:bool)
        n266 = Equal?(x=1.0, y=w535) -> (x = y?=w534:bool)
        n267 = Equal?(x=w540, y=w535) -> (x = y?=w530:bool)
        n268 = Equal?(x=w539, y=w535) -> (x = y?=w531:bool)
        n269 = Equal?(x=w538, y=w535) -> (x = y?=w532:bool)
        n270 = Equal?(x=w537, y=w535) -> (x = y?=w533:bool)
        n271 = case shown="False" w543 {
          tunnel: [FALSE TRUE] -> w542
          frame False {
            n272 = local write "SEGURIDAD"(TRUE ("SECUENCIA")) -> ()
          }
          frame True {
            w558 = FALSE ("ACTIVAR Campo")
            w556 = FALSE ("Bool3")
            n273 = local write "ACTIVAR ECRH"(w558) -> ()
            n274 = local write "ACTIVAR Campo"(w558) -> ()
            n275 = local write "INYECCION DE GAS"(w558) -> ()
            n276 = local write "Bool3"(w556) -> ()
            n277 = local write "Bool2"(w556) -> ()
            n278 = local write "Bool1"(w556) -> ()
            n279 = local write "Bool0"(w556) -> ()
            n280 = local write "SECUENCIA INICIADA"(w556) -> ()
            "SEGURIDAD" <- FALSE ("SECUENCIA")
            "SECUENCIA FINALIZADA" <- TRUE ("SECUENCIA FINALIZADA")
          }
        }
        n281 = case shown="False" w534 {
          frame False {
          }
          frame True {
            "SECUENCIA INICIADA" <- TRUE ("SECUENCIA INICIADA")
          }
        }
        n282 = case shown="False" w533 {
          frame False {
          }
          frame True {
            "Bool3" <- TRUE ("Bool3")
          }
        }
        n283 = case shown="False" w532 {
          frame False {
          }
          frame True {
            "Bool2" <- TRUE ("Bool2")
          }
        }
        n284 = case shown="True" "Stop Button" {
          frame False {
          }
          frame True {
            w548 = TRUE ("E. ECRH")
            "E. Campo" <- w548
            "E. ECRH" <- w548
          }
        }
        n285 = case shown="False" w531 {
          frame False {
          }
          frame True {
            "Bool1" <- TRUE ("Bool1")
          }
        }
        n286 = local read "Corriente"() -> (w524:dbl)
        n287 = Greater?(x=w524, y=900.0) -> (0:w527:bool)
        n288 = Less?(x=w524, y=650.0) -> (x < y?=w526:bool)
        n289 = case shown="True" w527 {
          frame False {
          }
          frame True {
            w547 = TRUE ("E. Campo")
            n290 = local write "E. Campo"(w547) -> ()
            n291 = local write "E. ECRH"(w547) -> ()
          }
        }
        n292 = case shown="False" w526 {
          frame False {
            n293 = local write "E. ECRH"(FALSE ("E. ECRH")) -> ()
          }
          frame True {
            n294 = local write "E. ECRH"(TRUE ("E. ECRH")) -> ()
          }
        }
        n295 = case shown="False" w530 {
          frame False {
          }
          frame True {
            "Bool0" <- TRUE ("Bool0")
          }
        }
        "Cuenta A" <- w535
      }
      n296 = timed-loop {
        tunnel: w363 -> [w594]
        timing-out: [_] -> w377
        timing: w378 -> [_]
        tunnel: w362 -> [w569]
        tunnel: w361 -> [w599]
        tunnel: w360 -> [w598]
        shift-right: [w595] -> _
        shift-left: 0 -> [w596]
        stop <- w606 stop-if-true
        # "Loop B-DATA LOG-"
        n297 = node-c288() -> (w597:i64)  [unwired: 1 in]
        "Iteration Duration B" <- w597
        n298 = flat-sequence {
          tunnel: w598 -> [w612]
          tunnel: w599 -> [w611]
          tunnel: [w610] -> w605
          tunnel: [w609] -> w604
          tunnel: [w608] -> w590
          tunnel: w605 -> [w629]
          tunnel: w604 -> [w628]
          tunnel: [w627] -> w603
          tunnel: [w626] -> w602
          tunnel: [w624] -> w591
          tunnel: w590 -> [w624]
          tunnel: [w625] -> w589
          tunnel: w603 -> [w651]
          tunnel: w602 -> [w650]
          tunnel: [w649] -> w601
          tunnel: [w648] -> w600
          tunnel: [w647] -> w592
          tunnel: w591 -> [w647]
          tunnel: w589 -> [w644]
          tunnel: [w646] -> w587
          tunnel: [w643] -> w585
          tunnel: w601 -> [w703]
          tunnel: w600 -> [w702]
          tunnel: [w701] -> w593
          tunnel: w592 -> [w701]
          tunnel: [w700] -> w588
          tunnel: w587 -> [w700]
          tunnel: [w699] -> w586
          tunnel: w585 -> [w699]
          tunnel: w593 -> [w718]
          tunnel: w588 -> [w717]
          tunnel: w586 -> [w716]
          tunnel: [w718] -> w584
          tunnel: [w717] -> w583
          tunnel: [w716] -> w582
          tunnel: [w714] -> w581
          tunnel: [w710] -> w580
          tunnel: [w708] -> w579
          tunnel: w584 -> [w808]
          tunnel: w583 -> [w807]
          tunnel: w582 -> [w806]
          tunnel: w581 -> [w805]
          tunnel: w580 -> [w804]
          tunnel: w579 -> [w803]
          tunnel: [w808] -> w578
          tunnel: [w807] -> w577
          tunnel: [w806] -> w576
          tunnel: [w805] -> w575
          tunnel: [w804] -> w574
          tunnel: [w803] -> w573
          tunnel: [w798] -> w572
          tunnel: [w795] -> w571
          tunnel: [w792] -> w570
          tunnel: w578 -> [w899]
          tunnel: w577 -> [w898]
          tunnel: w576 -> [w897]
          tunnel: w575 -> [w896]
          tunnel: w574 -> [w895]
          tunnel: w573 -> [w894]
          tunnel: w572 -> [w893]
          tunnel: w571 -> [w892]
          tunnel: w570 -> [w891]
          tunnel: w569 -> [w889]
          frame #0 {
            n299 = Concatenate Strings("#01RDCG1", "\r") -> (w617:string)
            n300 = VISA Write(VISA resource name=w611, write buffer=w617, error in (no error)=w612) -> (VISA resource name out=w621:refnum<visa-resource-name>, error out=w622:errorcluster)  [unwired: 1 out]
            n301 = VISA Read(VISA resource name=w621, byte count=13, error in (no error)=w622) -> (VISA resource name out=w610:refnum<visa-resource-name>, read buffer=w623:string, error out=w609:errorcluster)  [unwired: 1 out]
            n302 = Search/Split String(string=w623, search string/char (-)=" ", offset (0)=3) -> (match + rest of string=w614:string)  [unwired: 2 out]
            n303 = Fract/Exp String To Number(use system decimal point (T)=FALSE, string=w614) -> (number=w608:dbl)  [unwired: 2 in, 1 out]
            "CG1" <- w608
          }
          frame #1 {
            n304 = Concatenate Strings("#01RDCG2", "\r") -> (w636:string)
            n305 = VISA Write(VISA resource name=w629, write buffer=w636, error in (no error)=w628) -> (VISA resource name out=w639:refnum<visa-resource-name>, error out=w640:errorcluster)  [unwired: 1 out]
            n306 = VISA Read(VISA resource name=w639, byte count=13, error in (no error)=w640) -> (VISA resource name out=w627:refnum<visa-resource-name>, read buffer=w630:string, error out=w626:errorcluster)  [unwired: 1 out]
            n307 = Search/Split String(string=w630, search string/char (-)=" ", offset (0)=3) -> (match + rest of string=w634:string)  [unwired: 2 out]
            n308 = Fract/Exp String To Number(use system decimal point (T)=FALSE, string=w634) -> (number=w625:dbl)  [unwired: 2 in, 1 out]
            "CG2" <- w625
          }
          frame #2 {
            n309 = Concatenate Strings("#01RD", "\r") -> (w658:string)
            n310 = xnode "Set Dynamic Data Attributes"("Signals In"=w644, "Signal Name"="CG2") -> ("Signals Out"=w646:dynamicdata)  [unwired: 3 in, 1 out]
            n311 = VISA Write(VISA resource name=w651, write buffer=w658, error in (no error)=w650) -> (VISA resource name out=w661:refnum<visa-resource-name>, error out=w662:errorcluster)  [unwired: 1 out]
            n312 = VISA Read(VISA resource name=w661, byte count=13, error in (no error)=w662) -> (VISA resource name out=w649:refnum<visa-resource-name>, read buffer=w652:string, error out=w648:errorcluster)  [unwired: 1 out]
            n313 = Search/Split String(string=w652, search string/char (-)=" ", offset (0)=3) -> (match + rest of string=w656:string)  [unwired: 2 out]
            n314 = Fract/Exp String To Number(use system decimal point (T)=FALSE, string=w656) -> (number=w642:dbl)  [unwired: 2 in, 1 out]
            "IG" <- w642
            n315 = xnode "Set Dynamic Data Attributes"("Signals In"=w642, "Signal Name"="IG") -> ("Signals Out"=w643:dynamicdata)  [unwired: 3 in, 1 out]
          }
          frame #3 {
            n316 = VISA Flush I/O Buffer(VISA resource name=w703, error in (no error)=w702) -> (VISA resource name out=w705:refnum<visa-resource-name>, error out=w704:errorcluster)  [unwired: 1 in]
            n317 = VISA Close(VISA resource name=w705, error in (no error)=w704) -> ()  [unwired: 1 out]
          }
          frame #4 {
            n318 = call "DAQ Assistant"() -> ("data"=w732:dynamicdata)  [unwired: 17 in, 2 out]
            n319 = Split Signals(w732) -> (w722:dynamicdata, w721:dynamicdata, w720:dynamicdata)  [unwired: 3 in]
            n320 = Absolute Value(x=w722) -> (abs(x)=w736:dynamicdata)
            n321 = Multiply(x=w736, y=5419.3) -> (x*y=w734:dynamicdata)
            n322 = Subtract(x=w734, y=10.0) -> (x-y=w713:dynamicdata)
            "P. Forward" <- w713
            "Forward" <- w713
            n323 = xnode "Set Dynamic Data Attributes"("Signals In"=w713, "Signal Name"="P.Forward") -> ("Signals Out"=w714:dynamicdata)  [unwired: 3 in, 1 out]
            n324 = Absolute Value(x=w721) -> (abs(x)=w731:dynamicdata)
            n325 = Multiply(x=w731, y=2873.3) -> (x*y=w729:dynamicdata)
            n326 = To Single Precision Float(number=w720) -> (single precision float=w719:sgl)
            n327 = Subtract(x=w729, y=9.0) -> (x-y=w711:dynamicdata)
            "P. Reflected" <- w711
            "Reflected" <- w711
            n328 = Add(1:w711, 2:w713) -> (0:→"Total" →"Total":dynamicdata)  [unwired: 1 in, 1 out]
            n329 = Divide(x=w719, y=237.9) -> (x/y=w724:dbl)
            n330 = Subtract(x=w724, y=0.004) -> (x-y=w723:dbl)
            n331 = xnode "Set Dynamic Data Attributes"("Signals In"=w711, "Signal Name"="P.Reflected") -> ("Signals Out"=w710:dynamicdata)  [unwired: 3 in, 1 out]
            n332 = Multiply(x=w723, y=62500.0) -> (x*y=w706:dbl)
            "Corriente" <- w706
            "Corriente" <- w706
            n333 = xnode "Set Dynamic Data Attributes"("Signals In"=w706, "Signal Name"="Corriente") -> ("Signals Out"=w708:dynamicdata)  [unwired: 3 in, 1 out]
          }
          frame #5 {
            w800 = 100
            n334 = call "DAQ Assistant10"() -> ("data"=w825:dynamicdata)  [unwired: 17 in, 2 out]
            n335 = Split Signals(w825) -> (w814:dynamicdata, w813:dynamicdata, w812:dynamicdata)  [unwired: 3 in]
            n336 = Add(x=w813, y=0.0054) -> (x+y=w810:dynamicdata)
            n337 = Add(x=w812, y=0.005) -> (x+y=w811:dynamicdata)
            n338 = Add(x=w814, y=0) -> (x+y=w809:dynamicdata)
            n339 = Subtract(x=w810, y=1.25) -> (x-y=w822:dynamicdata)
            n340 = Subtract(x=w811, y=1.25) -> (x-y=w818:dynamicdata)
            n341 = Subtract(x=w809, y=1.25) -> (x-y=w827:dynamicdata)
            n342 = Divide(x=w818, y=0.005) -> (x/y=w793:dynamicdata)
            "Bobina 4" <- w793
            n343 = Divide(x=w822, y=0.005) -> (x/y=w796:dynamicdata)
            "Bobina 0" <- w796
            n344 = Divide(x=w827, y=0.005) -> (x/y=w799:dynamicdata)
            "Bobina 8" <- w799
            n345 = Greater?(x=w796, y=w800) -> (0:→"Boolean0":dynamicdata)
            n346 = Greater?(x=w799, y=w800) -> (0:→"Boolean8":dynamicdata)
            n347 = Greater?(x=w793, y=w800) -> (0:→"Boolean4":dynamicdata)
            n348 = xnode "Set Dynamic Data Attributes"("Signals In"=w796, "Signal Name"="T. Bobina 0") -> ("Signals Out"=w795:dynamicdata)  [unwired: 3 in, 1 out]
            n349 = xnode "Set Dynamic Data Attributes"("Signals In"=w799, "Signal Name"="T. Bobina 8") -> ("Signals Out"=w798:dynamicdata)  [unwired: 3 in, 1 out]
            n350 = xnode "Set Dynamic Data Attributes"("Signals In"=w793, "Signal Name"="T. Bobina 4") -> ("Signals Out"=w792:dynamicdata)  [unwired: 3 in, 1 out]
          }
          frame #6 {
            n351 = local read "Flujo"() -> (w884:dbl)
            n352 = local read "SP1"() -> (w887:dbl)
            n353 = xnode "Set Dynamic Data Attributes"("Signals In"=w884, "Signal Name"="Flujo") -> ("Signals Out"=w885:dynamicdata)  [unwired: 3 in, 1 out]
            n354 = xnode "Set Dynamic Data Attributes"("Signals In"=w887, "Signal Name"="SP") -> ("Signals Out"=w888:dynamicdata)  [unwired: 3 in, 1 out]
            n355 = Merge Signals(w899, w898, w897, w888, w885, w896, w895, w894, w893, w892, w891) -> (w890:dynamicdata)
            n356 = call "Write To Measurement File"("Signals"=w890, "Filename"=w889) -> ()  [unwired: 15 in, 3 out]
          }
        }
        n357 = Add(x=w597, y=w596) -> (x+y=w595:i64)
        "Cuenta B" <- w595
        n358 = Less?(x=w594, y=w595) -> (x < y?=w607:bool)
        n359 = case shown="False" w607 {
          tunnel: [FALSE TRUE] -> w606
          frame False {
            n360 = local write "DATOS"(TRUE ("SECUENCIA")) -> ()
          }
          frame True {
            "DATOS" <- FALSE ("SECUENCIA")
          }
        }
      }
      n361 = node-c288(w371) -> ()
      n362 = node-c288(w375) -> ()
      n363 = node-c288(w373) -> ()
      n364 = node-c288(w377) -> ()
    }
  }
